vi "medicaoIXV.vi"() -> ()   [LabVIEW 2012]
uses:
  <vilib>/Utility/file.llb/Write To Spreadsheet File (string).vi
  <vilib>/Utility/file.llb/Write To Spreadsheet File (DBL).vi
  <instrlib>/Agilent 6XXX Series/Agilent 6XXX Series.lvlib
  <vilib>/Analysis/NI_AALBase.lvlib
panel:
  out "stopLoopMedicoes":bool caption="Parar Medição"
  out "desvio":dbl format="%0.2f"
  out "reset graph":bool=TRUE
  out "tabela":dbl[][](array[numeric])
  in  "Tab Control":enum32{"Entrada de dados", "Saída de dados"}(tab)
  in  "Irradiância":dbl caption="Irradiância(W/cm²)"
  in  "nCurvas":i64=1 caption="Nº de curvas" min=1
  in  "T.J":dbl caption="Tensão\ndo joelho" step=0.1
  in  "p.a.j":dbl caption="Pontos antes\ndo joelho"
  in  "nMedições":i16=1 caption="N° medições por ponto" min=1
  in  "area":dbl caption="Área da célula(cm²)"
  in  "Tipo":string caption="Tipo da célula"
  in  "Formato":u16(ring) items=[".txt", ".csv"]
  out "ON/OFF1":bool caption="ON/OFF"
  in  "p.d.j":dbl caption="Pontos depois\ndo joelho"
  in  "T.M":dbl caption="Tensão máxima" step=0.1
  in  "Nome da célula":string
  in  "Local":path
  in  "Delay(ms)":dbl
  in  "Start":bool
  in  "temperatura":dbl caption="Temperatura da célula"
  in  "stopProgram":bool caption="Parar Programa"
  out "Imp":dbl caption="Imp(A)"
  out "Vmp":dbl caption="Vmp(V)"
  out "Pmp":dbl caption="Pmp(W)"
  out "Icc (A)":dbl
  out "Vca (V)":dbl
  in  "Print Screen":bool
  out "IXV":cluster{"Y":dbl[], "Y":dbl[]}[](graph)
  out "output voltage":dbl
  out "vAtual":dbl caption="Tensao Atual (V)"
  out "iAtual":dbl caption="Corrente Atual\n(A)"
  out "Ponto Atual":i32
  out "tabela":dbl[][](array[numeric]) caption="TABELA DE DADOS\nTensão(Fonte)      Pontos             Tensao           Corrente" format="%0.8f"
  in  "stop":bool caption="Parar Medição"
  out "ON/OFF2":bool caption="ON/OFF"
  out "eficiencia":dbl caption="Eficiencia(%)"
  out "FF":dbl
  in  "CorrenteGraph":dbl
  in  "TensaoGraph":dbl
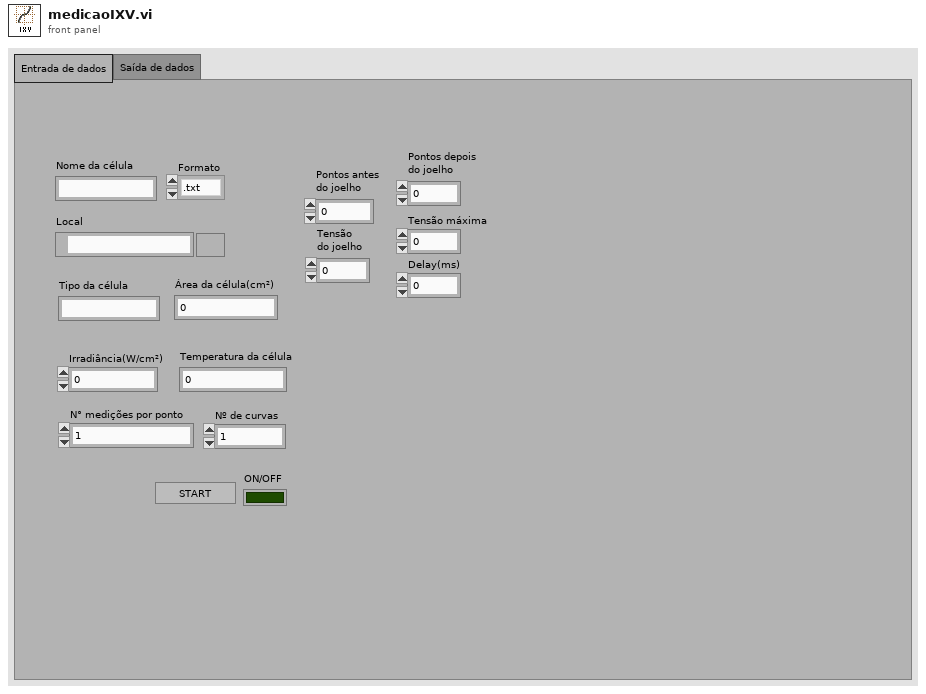
[diagram p1: front panel]
types:
  T1 = typedef "imagedata.ctl" = cluster{"image type":i32, "image depth":i32, "image":u8[], "mask":u8[], "colors":u32[], "Rectangle":cluster{"left":i16, "top":i16, "right":i16, "bottom":i16}}
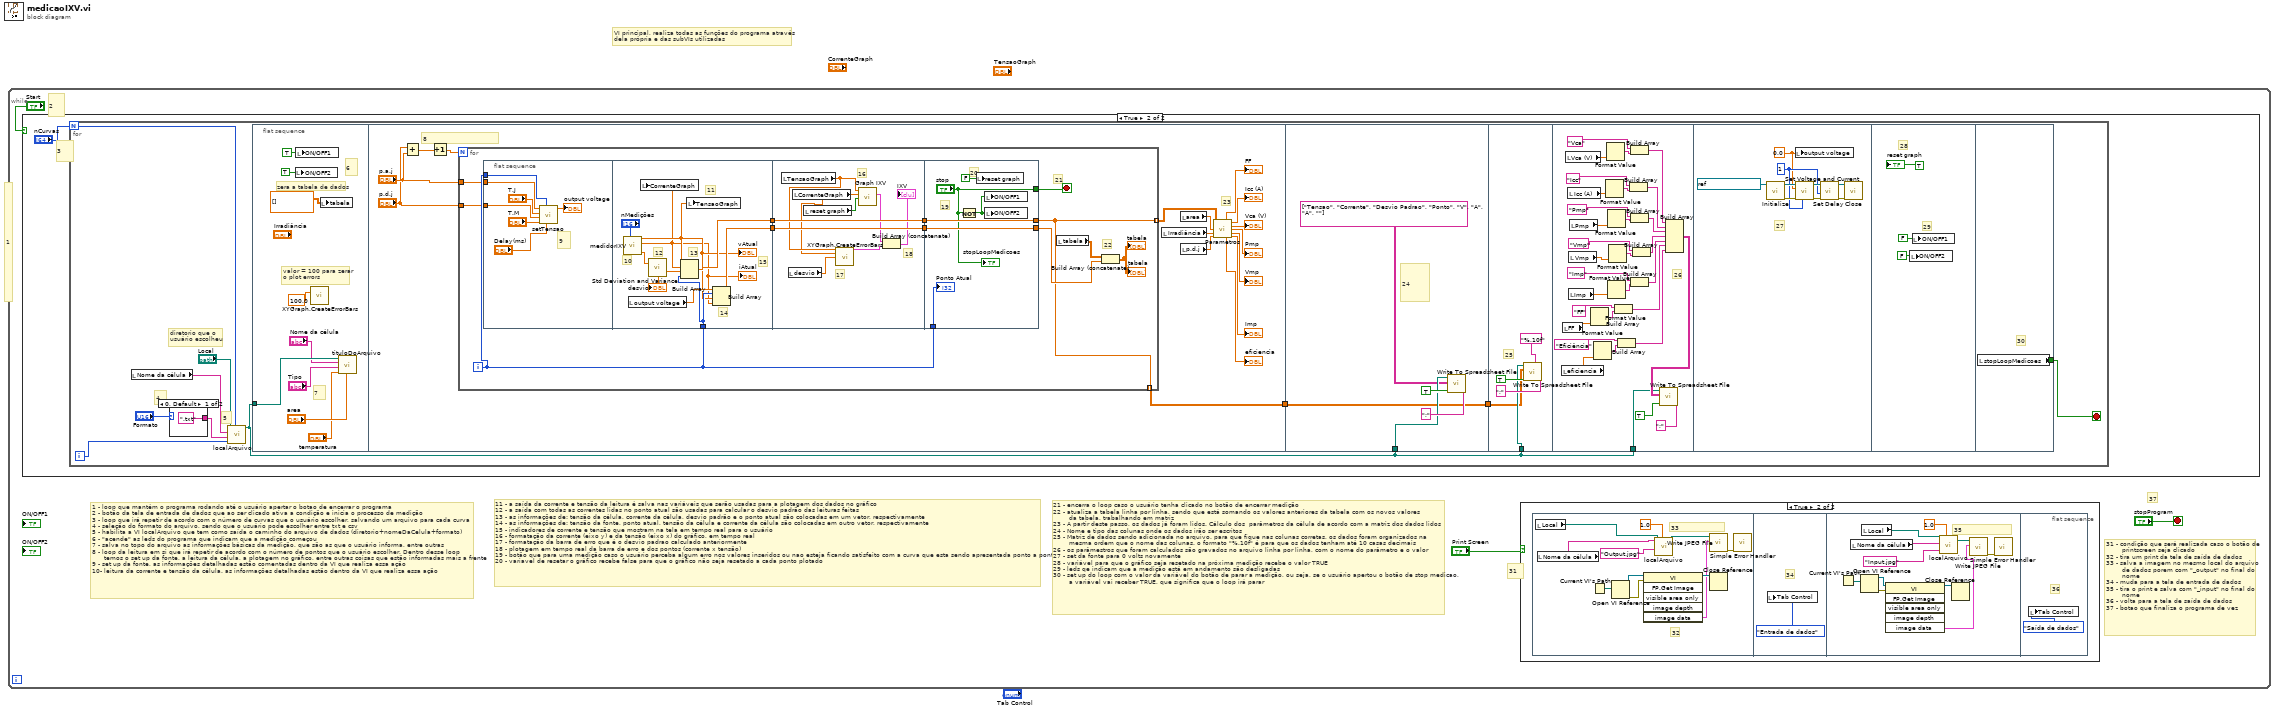
[diagram p0: block diagram]
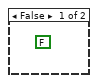
[diagram p3: hidden frame]
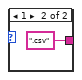
[diagram p4: hidden frame]
diagram:
  # "1"
  # "VI principal, realiza todas as funções do programa através \ndela própria e das subVIs utilizadas"
  n1 = while {
    stop <- "stopProgram" stop-if-true
    # "21 - encerra o loop caso o usuário tenha clicado no botão de encerrar medição\n22 - atualiza a tabela linha por linha, sendo que está somando os valores anteriores da tabela com os novos valores\n        da tabela, trabalhando em matriz\n23 - A partir deste passo, os dados já foram lidos. Cálculo dos  parâmetros da célula de acordo com a matriz dos dados lidos\n24 - Nome e tipo das colunas onde os dados irão ser escritos\n25 - Matriz de dados sendo adicionada no arquivo. para que fique nas colunas corretas, os dados foram organizados na \n        mesma ordem que o nome das colunas. o formato \"%.10f\" é para que os dados tenham até 10 casas decimais\n26 - os parâmestros que foram calculados são gravados no arquivo linha por linha, com o nome do parâmetro e o valor\n27 - set da fonte para 0 volts novamente \n28 - variável para que o gráfico seja resetado na próxima medição recebe o valor TRUE \n29 - leds qe indicam que a medição está em andamento são desligadas\n30 - set up do loop com o valor da variável do botão de parar a medição, ou seja, se o usuário apertou o botão de stop medicao,\n        a variável vai receber TRUE, que significa que o loop irá parar"
    # "11 - a saída da corrente e tensão da leitura é salva nas variáveis que serão usadas para a plotagem dos dados no gráfico\n12 - a saída com todas as correntes lidas no ponto atual são usadas para calcular o desvio padrão das leituras feitas\n13 - as informações de: tensão da célula, corrente da célula, desvio padrão e o ponto atual são colocadas em um vetor, respectivamente\n14 - as informações de: tensão da fonte, ponto atual, tensão da célula e corrente da célula são colocadas em outro vetor, respectivamente\n15 - indicadores de corrente e tensão que mostram na tela em tempo real para o usuário \n16 - formatação da corrente (eixo y) e da tensão (eixo x) do gráfico, em tempo real\n17 - formatação da barra de erro que é o desvio padrao calculado anteriormente\n18 - plotagem em tempo real da barra de erro e dos pontos (corrente x tensão)\n19 - botão que para uma medição caso o usuário perceba algum erro nos valores inseridos ou nao esteja ficando satisfeito com a curva que esta sendo apresentada ponto a ponto\n20 - variavel de resetar o gráfico recebe false para que o gráfico não seja resetado a cada ponto plotado"
    # "1 - loop que mantém o programa rodando até o usuário apertar o botao de encerrar o programa\n2 - botão da tela de entrada de dados que ao ser clicado ativa a condição e inicia o processo de medição\n3 - loop que irá repetir de acordo com o número de curvas que o usuário escolher, salvando um arquivo para cada curva \n4 - seleção do formato do arquivo, sendo que o usuário pode escolher entre txt e csv\n5 - habilita a VI localArquivo que tem como saída o caminho do arquivo de dados (diretorio+nomeDaCelula+formato) \n6 - \"acende\" as leds do programa que indicam que a medição começou\n7 - salva no topo do arquivo as informações básicas da medição, que são as que o usuário informa, entre outras\n8 - loop da leitura em si que irá repetir de acordo com o número de pontos que o usuário escolher. Dentro desse loop\n      temos o set up da fonte, a leitura da célula, a plotagem no gráfico, entre outras coisas que estão informadas mais a frente\n9 - set up da fonte, as informações detalhadas estão comentadas dentro da VI que realiza essa ação\n10- leitura da corrente e tensão da célula. as informações detalhadas estão dentro da VI que realiza essa ação"
    # "31 - condição que será realizada caso o botão de\n        printscreen seja clicado\n32 - tira um print da tela de saída de dados\n33 - salva a imagem no mesmo local do arquivo\n        de dados porem com \"_output\" no final do\n        nome\n34 - muda para a tela de entrada de dados\n35 - tira o print e salva com \"_input\" no final do\n        nome\n36 - volta para a tela de saída de dados \n37 - botao que finaliza o programa de vez"
    # "37"
    # "31"
    # "2"
    n2 = case shown="True" "Start" {
      frame False {
        (unwired) FALSE
      }
      frame True {
        # "3"
        n3 = for {
          N: "nCurvas" -> [w31]
          i -> [w30]
          stop <- w29 stop-if-true
          # "diretorio que o\nusuário escolheu"
          # "5"
          # "4"
          n4 = local read "Nome da célula"() -> (w34:string)
          n5 = case shown="0, Default" "Formato" {
            tunnel: [".txt" ".csv"] -> w33
            frame 0, Default {
            }
            frame 1 {
            }
          }
          n6 = call "localArquivo.vi"("quantidadeDeArquivos"=w31, "nAtualDoArquivo"=w30, "extensão"=w33, "Nome do arquivo"=w34, "Local"="Local") -> ("Path"=w32:path)  [unwired: 6 in]
          n7 = flat-sequence {
            tunnel: w32 -> [w49]
            tunnel: [w61] -> w38
            tunnel: w32 -> [w111]
            tunnel: [w110] -> w37
            tunnel: w38 -> [w110]
            tunnel: w32 -> [w115]
            tunnel: w37 -> [w114]
            tunnel: w32 -> [w127]
            tunnel: [w163] -> w29
            frame #0 {
              # "zera a tabela de dados"
              # "7"
              # "6"
              # "valor = 100 para zerar\no plot errors"
              n8 = local write "ON/OFF2"(TRUE ("ON/OFF2")) -> ()
              n9 = local write "ON/OFF1"(TRUE ("ON/OFF")) -> ()
              n10 = call "XYGraph.CreateErrorBars.vi"("yTemp"=100.0) -> ()  [unwired: 14 in, 1 out]
              n11 = local write "tabela"(dbl[][] [] ("array")) -> ()
              n12 = call "tituloDoArquivo.vi"("area"="area", "temperatura"="temperatura", "Tipo"="Tipo", "Nome da célula"="Nome da célula", "file path (dialog if empty)"=w49) -> ()  [unwired: 7 in]
            }
            frame #1 {
              # "23"
              # "8"
              n13 = Add(x="p.d.j", y="p.a.j") -> (x+y=w64:dbl)
              n14 = Increment(x=w64) -> (x+1=w65:dbl)
              n15 = for {
                N: w65 -> [_]
                tunnel: [w66] -> w54 mode=indexing
                tunnel: "p.a.j" -> [w68]
                tunnel: "p.d.j" -> [w67]
                tunnel: [w66] -> w61 mode=indexing
                i -> [w72]
                stop <- w71 stop-if-true
                # "22"
                # "21"
                n16 = flat-sequence {
                  tunnel: w72 -> [w83]
                  tunnel: w68 -> [w81]
                  tunnel: w67 -> [w80]
                  tunnel: w72 -> [w89]
                  tunnel: [w91] -> w77
                  tunnel: [w93] -> w76
                  tunnel: [w102] -> w70
                  tunnel: [w101] -> w69
                  tunnel: w76 -> [w101]
                  tunnel: w77 -> [w102]
                  tunnel: [w107] -> w75
                  tunnel: [w108] -> w66
                  tunnel: w70 -> [w108]
                  tunnel: w69 -> [w107]
                  tunnel: w72 -> [w106]
                  tunnel: ["stop"] -> w71
                  frame #0 {
                    # "9"
                    n17 = call "setTensao.vi"("delay(ms)"="Delay(ms)", "Ponto atual"=w83, "T.M"="T.M", "P.D.J"=w80, "T.J"="T.J", "P.A.J"=w81) -> ("output voltage"=→"output voltage":dbl)  [unwired: 5 in]
                  }
                  frame #1 {
                    # "15"
                    # "14"
                    # "13"
                    # "11"
                    # "12"
                    # "10"
                    n18 = call "medidorIXV.vi"("nMedicoes"="nMedições") -> ("Tensao Atual"=w88:dbl, "Corrente Atual"=w87:dbl, "vetorCorrente"=w90:dbl[])  [unwired: 7 in]
                    "iAtual" <- w87
                    "vAtual" <- w88
                    n19 = local read "output voltage"() -> (w92:dbl)
                    n20 = local write "CorrenteGraph"(w87) -> ()
                    n21 = call <vilib>:"Std Deviation and Variance.vi"("X"=w90) -> ("standard deviation"=w86:dbl)  [unwired: 1 in, 2 out]
                    "desvio" <- w86
                    n22 = Build Array(w88, w87, w86, w89) -> (w91:dbl[])
                    n23 = local write "TensaoGraph"(w88) -> ()
                    n24 = Build Array(w92, w89, w88, w87) -> (w93:dbl[])
                  }
                  frame #2 {
                    # "17"
                    # "18"
                    # "16"
                    n25 = local read "TensaoGraph"() -> (w96:dbl)
                    n26 = local read "desvio"() -> (w94:dbl)
                    n27 = local read "CorrenteGraph"() -> (w95:dbl)
                    n28 = local read "reset graph"() -> (w100:bool)
                    n29 = call "XYGraph.CreateErrorBars.vi"("xTemp"=w96, "yTemp"=w95, "errorTemp"=w94) -> ("error bar plot"=w97:cluster{dbl[], dbl[]})  [unwired: 12 in]
                    n30 = call "Graph IXV"("Reset"=w100, "Y Input"=w95, "X Input"=w96) -> ("XY Graph"=w99:cluster{"Y":dbl[], "Y":dbl[]}[])  [unwired: 2 in, 6 out]
                    n31 = Build Array (concatenate)(w99, w97) -> (→"IXV":cluster{"Y":dbl[], "Y":dbl[]}[])
                  }
                  frame #3 {
                    # "20"
                    # "19"
                    n32 = Not(x="stop") -> (.not. x?=w104:bool)
                    n33 = local write "reset graph"(FALSE) -> ()
                    n34 = local write "ON/OFF1"(w104) -> ()
                    n35 = local write "ON/OFF2"(w104) -> ()
                    "Ponto Atual" <- w106
                    "stopLoopMedicoes" <- "stop"
                  }
                }
                n36 = local read "tabela"() -> (w74:dbl[][])
                n37 = Build Array (concatenate)(w74, w75) -> (→"tabela" →"tabela":dbl[][])
              }
              n38 = local read "Irradiância"() -> (w52:dbl)
              n39 = local read "area"() -> (w53:dbl)
              n40 = local read "p.d.j"() -> (w55:dbl)
              n41 = call "Parametros.vi"("VetorDeDados"=w54, "area"=w53, "irradiancia"=w52, "pontos"=w55) -> ("FF"=→"FF":dbl, "Icc"=→"Icc (A)":dbl, "Vca"=→"Vca (V)":dbl, "Pmp"=→"Pmp":dbl, "Vmp"=→"Vmp":dbl, "eficiencia"=→"eficiencia":dbl, "Imp"=→"Imp":dbl)  [unwired: 5 in]
            }
            frame #2 {
              # "24"
              n42 = call-poly <vilib>:"Write To Spreadsheet File.vi"("delimiter (\\t)"=";" ("delimiter (\\t)"), "append to file? (new file:F)"=TRUE, "2D data"=string[][] [["Tensao", "Corrente", "Desvio Padrao", "Ponto"], ["V", "A", "A", ""]], "file path (dialog if empty)"=w111) -> ()  [unwired: 4 in, 1 out]
            }
            frame #3 {
              # "25"
              n43 = call-poly <vilib>:"Write To Spreadsheet File.vi"("delimiter (\\t)"=";" ("delimiter (\\t)"), "format (%.3f)"="%.10f", "append to file? (new file:F)"=TRUE, "2D data"=w114, "file path (dialog if empty)"=w115) -> ()  [unwired: 3 in, 1 out]
            }
            frame #4 {
              # "26"
              n44 = local read "eficiencia"() -> (w121:dbl)
              n45 = local read "FF"() -> (w122:dbl)
              n46 = local read "Vca (V)"() -> (w129:dbl)
              n47 = local read "Icc (A)"() -> (w139:dbl)
              n48 = local read "Imp"() -> (w142:dbl)
              n49 = local read "Vmp"() -> (w141:dbl)
              n50 = local read "Pmp"() -> (w140:dbl)
              n51 = Format Value(value (0)=w122) -> (output string=w126:string)  [unwired: 2 in]
              n52 = Format Value(value (0)=w121) -> (output string=w125:string)  [unwired: 2 in]
              n53 = Format Value(value (0)=w139) -> (output string=w132:string)  [unwired: 2 in]
              n54 = Format Value(value (0)=w129) -> (output string=w130:string)  [unwired: 2 in]
              n55 = Format Value(value (0)=w140) -> (output string=w134:string)  [unwired: 2 in]
              n56 = Format Value(value (0)=w142) -> (output string=w138:string)  [unwired: 2 in]
              n57 = Format Value(value (0)=w141) -> (output string=w136:string)  [unwired: 2 in]
              n58 = Build Array("FF" ("string (\"\")"), w126) -> (w124:string[])
              n59 = Build Array("Eficiência" ("string (\"\")"), w125) -> (w123:string[])
              n60 = Build Array("Icc", w132) -> (w144:string[])
              n61 = Build Array("Vca", w130) -> (w143:string[])
              n62 = Build Array("Pmp", w134) -> (w145:string[])
              n63 = Build Array("Imp", w138) -> (w147:string[])
              n64 = Build Array("Vmp", w136) -> (w146:string[])
              n65 = Build Array(w143, w144, w145, w146, w147, w124, w123) -> (w148:string[][])
              n66 = call-poly <vilib>:"Write To Spreadsheet File.vi"("delimiter (\\t)"=";" ("delimiter (\\t)"), "append to file? (new file:F)"=TRUE, "2D data"=w148, "file path (dialog if empty)"=w127) -> ()  [unwired: 4 in, 1 out]
            }
            frame #5 {
              w151 = 0.0 ("voltage (0 V)")
              w154 = u8 1 ("channel (1)")
              # "27"
              n67 = call <instrlib>:"Initialize.vi"("VISA resource name"=refnum<visa-resource-name> "GPIB0::5::INSTR") -> ("error out"=w156:errorcluster, "VISA resource name out"=w155:refnum<visa-resource-name>)  [unwired: 9 in]
              n68 = local write "output voltage"(w151) -> ()
              n69 = call <instrlib>:"Set Voltage and Current.vi"("channel (1)"=w154, "error in (no error)"=w156, "voltage (0 V)"=w151, "VISA resource name"=w155) -> ("error out"=w157:errorcluster, "VISA resource name out"=w158:refnum<visa-resource-name>)  [unwired: 6 in]
              n70 = call <instrlib>:"Set Delay.vi"("error in (no error)"=w157, "channel (1)"=w154, "VISA resource name"=w158) -> ("error out"=w152:errorcluster, "VISA resource name out"=w153:refnum<visa-resource-name>)  [unwired: 7 in]
              n71 = call <instrlib>:"Close.vi"("error in (no error)"=w152, "VISA resource name"=w153) -> ()  [unwired: 9 in, 1 out]
            }
            frame #6 {
              # "29"
              # "28"
              n72 = local write "ON/OFF2"(FALSE ("ON/OFF")) -> ()
              n73 = local write "ON/OFF1"(FALSE) -> ()
              "reset graph" <- TRUE
            }
            frame #7 {
              # "30"
              n74 = local read "stopLoopMedicoes"() -> (w163:bool)
            }
          }
        }
      }
    }
    n75 = case shown="True" "Print Screen" {
      frame False {
      }
      frame True {
        n76 = flat-sequence {
          frame #0 {
            # "33"
            # "32"
            n77 = local read "Local"() -> (w7:path)
            n78 = local read "Nome da célula"() -> (w5:string)
            n79 = Current VI's Path() -> (path=w12:path)
            n80 = Open VI Reference(vi path=w12) -> (vi reference=w13:refnum<vi>, error out=w14:errorcluster)  [unwired: 5 in]
            n81 = invoke class="VI" method="FP.Get Image"(reference=w13, error in=w14) -> (reference out=w11:refnum<vi>, "image data"=w10:T1)  [unwired: 4 in, 4 out]
            n82 = call "localArquivo.vi"("quantidadeDeArquivos"=1.0, "extensão"="Output.jpg", "Nome do arquivo"=w5, "Local"=w7) -> ("Path"=w4:path)  [unwired: 7 in]
            n83 = call <vilib>:"Write JPEG File.vi"("image data"=w10, "path to JPEG file"=w4) -> ("error out"=w9:errorcluster)  [unwired: 8 in, 1 out]
            n84 = Close Reference(reference=w11) -> ()  [unwired: 1 in, 1 out]
            n85 = call <vilib>:"Simple Error Handler.vi"("error in (no error)"=w9) -> ()  [unwired: 4 in, 5 out]
          }
          frame #1 {
            # "34"
            n86 = local write "Tab Control"(enum32{"Entrada de dados", "Saída de dados"}."Entrada de dados" ("Tab Control")) -> ()
          }
          frame #2 {
            # "35"
            n87 = Current VI's Path() -> (path=w25:path)
            n88 = local read "Nome da célula"() -> (w19:string)
            n89 = Open VI Reference(vi path=w25) -> (vi reference=w24:refnum<vi>, error out=w23:errorcluster)  [unwired: 5 in]
            n90 = local read "Local"() -> (w18:path)
            n91 = invoke class="VI" method="FP.Get Image"(reference=w24, error in=w23) -> (reference out=w26:refnum<vi>, "image data"=w21:T1)  [unwired: 4 in, 4 out]
            n92 = call "localArquivo.vi"("quantidadeDeArquivos"=1.0, "extensão"="Input.jpg", "Nome do arquivo"=w19, "Local"=w18) -> ("Path"=w17:path)  [unwired: 7 in]
            n93 = Close Reference(reference=w26) -> ()  [unwired: 1 in, 1 out]
            n94 = call <vilib>:"Write JPEG File.vi"("image data"=w21, "path to JPEG file"=w17) -> ("error out"=w22:errorcluster)  [unwired: 8 in, 1 out]
            n95 = call <vilib>:"Simple Error Handler.vi"("error in (no error)"=w22) -> ()  [unwired: 4 in, 5 out]
          }
          frame #3 {
            # "36"
            n96 = local write "Tab Control"(enum32{"Entrada de dados", "Saída de dados"}."Saída de dados" ("Tab Control")) -> ()
          }
        }
      }
    }
  }
